vi "GetStepScript.vi"(8 "error in (no error)":errorcluster) -> (0 "error out":errorcluster, 2 "found":bool, 3 "StepScript":T1[](array[typedef]))   [LabVIEW 2016, in "SeqProcessor.lvlib"]
uses:
  SeqProcessor.lvlib
  controls/Step.ctl
  controls/StepType.ctl
  <vilib>/addons/PointValueMap/subVIs/Point_Read_variant.vi
  <vilib>/addons/PointValueMap/PointValueMap.lvlib
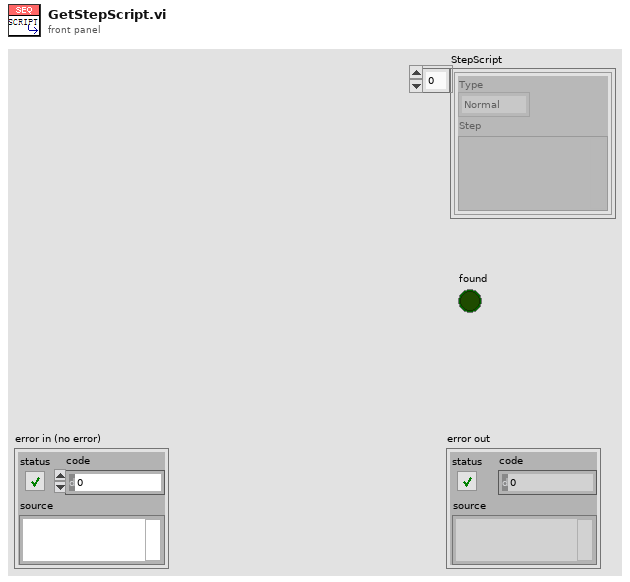
[diagram p1: front panel]
types:
  T1 = typedef "SeqProcessor.lvlib/Step.ctl" = cluster{"Type":T2, "Step":variant}
  T2 = typedef "SeqProcessor.lvlib/StepType.ctl" = enum16{"Normal", "Parallel", "Conditional", "Jump"}
  T3 = typedef "PointValueMap.lvlib/PointMap.ctl" = refnum<data-value>
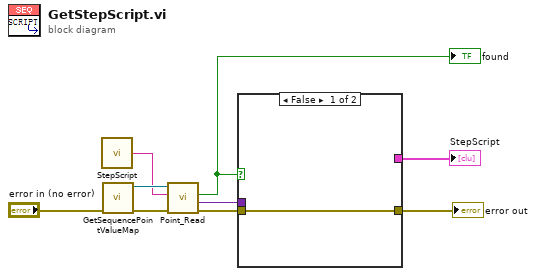
[diagram p0: block diagram]
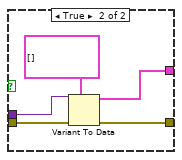
[diagram p2: hidden frame]
diagram:
  n1 = call "StepScript.vi"() -> ("StepScript"=w2:string)  [unwired: 5 in]
  n2 = call "GetSequencePointValueMap.vi"("error in (no error)"="error in (no error)") -> ("error out"=w5:errorcluster, "SeqMap"=w4:T3)  [unwired: 9 in]
  n3 = call-poly <vilib>:"Point_Read.vi"("Error In"=w5, "Tag"=w2, "Map"=w4) -> ("Error Out"=w8:errorcluster, "Value"=w7:variant, "Found?"=w6:bool)  [unwired: 3 in, 3 out]
  "found" <- w6
  n4 = case shown="False" w6 {
    tunnel: w8 -> [w10 w15]
    tunnel: [w10 w14] -> w3
    tunnel: w7 -> [_ w13]
    tunnel: [_ w12] -> w1
    frame False {
    }
    frame True {
      n5 = Variant To Data(error in=w15, type=T1[] [], Variant=w13) -> (data=w12:T1[], error out=w14:errorcluster)
    }
  }
  "error out" <- w3
  "StepScript" <- w1
